vi "Delete Block Diagram.vi"(8 "error in (no error)":errorcluster, 11 "VI Path":path) -> (0 "error out":errorcluster)   [LabVIEW 2020]
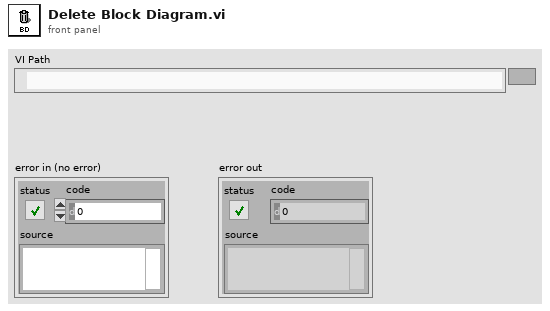
[diagram p1: front panel]
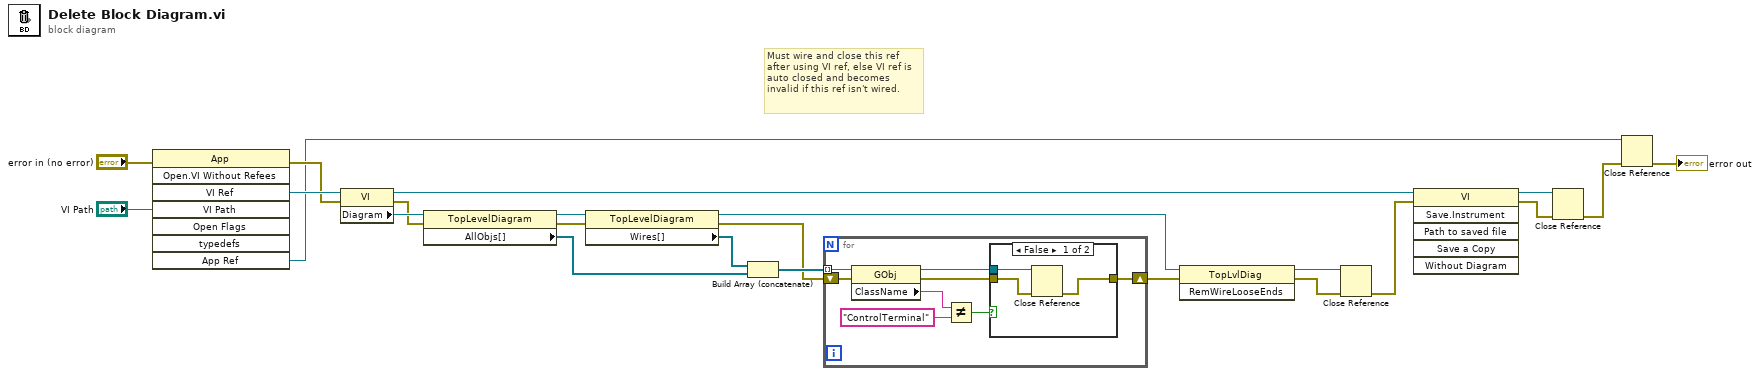
[diagram p0: block diagram]
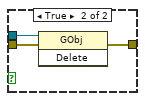
[diagram p2: hidden frame]
diagram:
  # "Must wire and close this ref after using VI ref, else VI ref is auto closed and becomes invalid if this ref isn't wired."
  n1 = invoke class="App" method="Open.VI Without Refees"(error in="error in (no error)", "VI Path"="VI Path") -> (error out=w6:errorcluster, "VI Ref"=w7:refnum<vi>, "App Ref"=w4:refnum<vi>)  [unwired: 6 in, 5 out]
  n2 = property class="VI"(reference=w7, error in=w6) -> (reference out=w20:refnum<vi>, error out=w13:errorcluster, "Diagram"=w15:refnum<vi>)
  n3 = property class="TopLevelDiagram"(reference=w15, error in=w13) -> (reference out=w12:refnum<vi>, error out=w14:errorcluster, "AllObjs[]"=w8:refnum<vi>[])
  n4 = property class="TopLevelDiagram"(reference=w12, error in=w14) -> (reference out=w11:refnum<vi>, error out=w9:errorcluster, "Wires[]"=w16:refnum<vi>[])
  n5 = Build Array (concatenate)(w16, w8) -> (w10:refnum<vi>[])
  n6 = for {
    tunnel: w10 -> [w31] mode=indexing
    shift-right: [w24] -> w23
    shift-left: w9 -> [w30]
    n7 = property class="GObj"(reference=w31, error in=w30) -> (reference out=w26:refnum<vi>, error out=w25:errorcluster, "ClassName"=w29:string)
    n8 = Not Equal?(x=w29, y="ControlTerminal") -> (x != y?=w27:bool)
    n9 = case shown="False" w27 {
      tunnel: w26 -> [w34 w37]
      tunnel: w25 -> [w33 w36]
      tunnel: [w32 w35] -> w24
      frame False {
        n10 = Close Reference(reference=w34, error in (no error)=w33) -> (error out=w32:errorcluster)
      }
      frame True {
        n11 = invoke class="GObj" method="Delete"(reference=w37, error in=w36) -> (error out=w35:errorcluster)  [unwired: 1 in, 2 out]
      }
    }
  }
  n12 = invoke class="TopLvlDiag" method="RemWireLooseEnds"(reference=w11, error in=w23) -> (reference out=w22:refnum<vi>, error out=w21:errorcluster)  [unwired: 1 in, 1 out]
  n13 = Close Reference(reference=w22, error in (no error)=w21) -> (error out=w19:errorcluster)
  n14 = invoke class="VI" method="Save.Instrument"(reference=w20, error in=w19) -> (reference out=w17:refnum<vi>, error out=w18:errorcluster)  [unwired: 4 in, 4 out]
  n15 = Close Reference(reference=w17, error in (no error)=w18) -> (error out=w5:errorcluster)
  n16 = Close Reference(reference=w4, error in (no error)=w5) -> (error out=→"error out":errorcluster)
